vi "Multi-Acq.vi"(8 "error in":errorcluster, 11 "Synapse CCD.lvclass In":refnum<class "Synapse CCD.lvclass">) -> (0 "error out":errorcluster, 2 "max value":i32, 3 "Synapse CCD.lvclass Out":refnum<class "Synapse CCD.lvclass">)   [LabVIEW 2017, in "Synapse CCD.lvclass"]
doc: "Perform multiple CCD acquisitions in succession.\nUse Setup Multi Acq.vi to properly setup multiple acquisitions."
uses:
  Synapse CCD.lvclass
  Synapse CCD.lvclass/Synapse CCD.ctl
panel:
  out "where ami":string
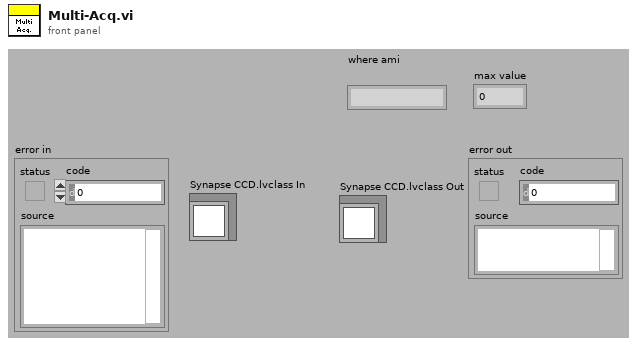
[diagram p1: front panel]
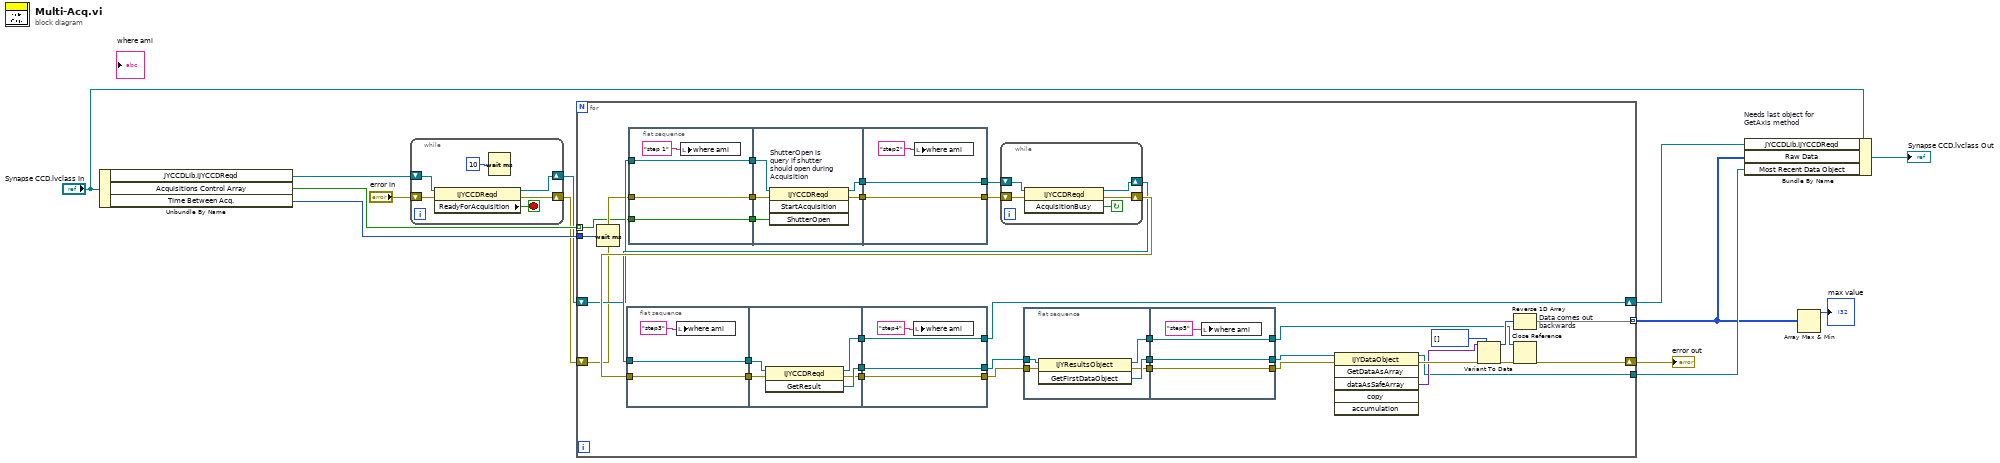
[diagram p0: block diagram]
diagram:
  n1 = Unbundle By Name("Synapse CCD.lvclass In") -> ("JYCCDLib.IJYCCDReqd"=w4:refnum<k7>, "Acquisitions Control Array"=w10:bool[], "Time Between Acq."=w9:u32)
  n2 = while {
    shift-right: [w18] -> w6
    shift-left: w4 -> [w19]
    shift-right: [w16] -> w5
    shift-left: "error in" -> [w17]
    stop <- w15 stop-if-true
    n3 = property class="IJYCCDReqd"(reference=w19, error in=w17) -> (reference out=w18:refnum<k7>, error out=w16:errorcluster, "ReadyForAcquisition"=w15:bool)
    n4 = Wait (ms)(milliseconds to wait=u32 10) -> ()  [unwired: 1 out]
  }
  n5 = for {
    shift-right: [w37] -> w13
    shift-left: w5 -> [w49]
    shift-right: [w48] -> w1
    shift-left: w6 -> [w50]
    tunnel: w10 -> [w47] mode=indexing
    tunnel: [w39] -> w3 mode=indexing
    tunnel: w9 -> [w35]
    tunnel: [w33] -> w8
    n6 = Wait (ms)(milliseconds to wait=w35) -> ()  [unwired: 1 out]
    n7 = flat-sequence {
      tunnel: w51 -> [w65]
      tunnel: w52 -> [w66]
      tunnel: [w66] -> w27
      tunnel: [w65] -> w26
      tunnel: w27 -> [w71]
      tunnel: w26 -> [w70]
      tunnel: [w69] -> w25
      tunnel: [w68] -> w24
      tunnel: [w67] -> w23
      tunnel: [w73] -> w45
      tunnel: [w74] -> w46
      tunnel: [w75] -> w48
      tunnel: w25 -> [w75]
      tunnel: w24 -> [w74]
      tunnel: w23 -> [w73]
      frame #0 {
        n8 = local write "where ami"("step3" ("where ami")) -> ()
      }
      frame #1 {
        n9 = invoke class="IJYCCDReqd" method="GetResult"(reference=w70, error in=w71) -> (reference out=w69:refnum<k7>, error out=w67:errorcluster, "GetResult"=w68:refnum<k7>)  [unwired: 1 in]
      }
      frame #2 {
        n10 = local write "where ami"("step4" ("where ami")) -> ()
      }
    }
    n11 = flat-sequence {
      tunnel: w47 -> [w77]
      tunnel: w49 -> [w78]
      tunnel: w50 -> [w79]
      tunnel: [w79] -> w32
      tunnel: [w78] -> w31
      tunnel: [w77] -> w30
      tunnel: w32 -> [w82]
      tunnel: w31 -> [w81]
      tunnel: w30 -> [w80]
      tunnel: [w84] -> w29
      tunnel: [w83] -> w28
      tunnel: [w86] -> w53
      tunnel: [w87] -> w54
      tunnel: w29 -> [w87]
      tunnel: w28 -> [w86]
      frame #0 {
        n12 = local write "where ami"("step 1" ("where ami")) -> ()
      }
      frame #1 {
        n13 = invoke on="ShutterOpen is \nquery if shutter\nshould open during\nAcquisition" class="IJYCCDReqd" method="StartAcquisition"(reference=w82, error in=w81, "ShutterOpen"=w80) -> (reference out=w84:refnum<k7>, error out=w83:errorcluster)  [unwired: 1 in, 2 out]
      }
      frame #2 {
        n14 = local write "where ami"("step2" ("where ami")) -> ()
      }
    }
    n15 = while {
      shift-right: [w88] -> w52
      shift-left: w53 -> [w89]
      shift-right: [w90] -> w51
      shift-left: w54 -> [w91]
      stop <- w92 continue-if-true
      n16 = invoke class="IJYCCDReqd" method="AcquisitionBusy"(reference=w91, error in=w89) -> (reference out=w90:refnum<k7>, error out=w88:errorcluster, "AcquisitionBusy"=w92:bool)  [unwired: 1 in]
    }
    n17 = flat-sequence {
      tunnel: w46 -> [w59]
      tunnel: w45 -> [w58]
      tunnel: [w57] -> w22
      tunnel: [w56] -> w21
      tunnel: [w55] -> w20
      tunnel: [w61] -> w36
      tunnel: [w62] -> w38
      tunnel: [w63] -> w40
      tunnel: w22 -> [w63]
      tunnel: w21 -> [w62]
      tunnel: w20 -> [w61]
      frame #0 {
        n18 = invoke class="IJYResultsObject" method="GetFirstDataObject"(reference=w59, error in=w58) -> (reference out=w55:refnum<k7>, error out=w56:errorcluster, "GetFirstDataObject"=w57:refnum<k7>)  [unwired: 1 in]
      }
      frame #1 {
        n19 = local write "where ami"("step5" ("where ami")) -> ()
      }
    }
    n20 = invoke class="IJYDataObject" method="GetDataAsArray"(reference=w40, error in=w38) -> (reference out=w33:refnum<k7>, error out=w43:errorcluster, "dataAsSafeArray"=w41:variant)  [unwired: 4 in, 3 out]
    n21 = Variant To Data(error in=w43, type=i32[] [], Variant=w41) -> (data=w44:i32[], error out=w34:errorcluster)
    n22 = Reverse 1D Array "Data comes out backwards"(array=w44) -> (reversed array=w39:i32[])
    n23 = Close Reference(reference=w36, error in (no error)=w34) -> (error out=w37:errorcluster)
  }
  "error out" <- w13
  n24 = Bundle By Name "Needs last object for GetAxis method"(cluster="Synapse CCD.lvclass In", "JYCCDLib.IJYCCDReqd"=w1, "Raw Data"=w3, "Most Recent Data Object"=w8) -> (→"Synapse CCD.lvclass Out":refnum<class "Synapse CCD.lvclass">)
  n25 = Array Max & Min(array=w3) -> (max value=→"max value":i32)  [unwired: 3 out]
